vi "FTW-Socket-Bind.vi"(0 "FTW Endpoint":refnum<class "FTW-Socket.lvclass">, 5 "Remote Endpoint Address":string, 11 "error in":errorcluster) -> (4 "FTW Endpoint out":refnum<class "FTW-Socket.lvclass">, 6 "Actual Endpoint Address":string, 15 "error out":errorcluster)   [LabVIEW 2013, in "FTW-Socket.lvclass"]
uses:
  FTW-Socket.lvclass
  FTW-Socket.lvclass/FTW-Socket.ctl
panel:
  # "Inputs"
  # "Outputs"
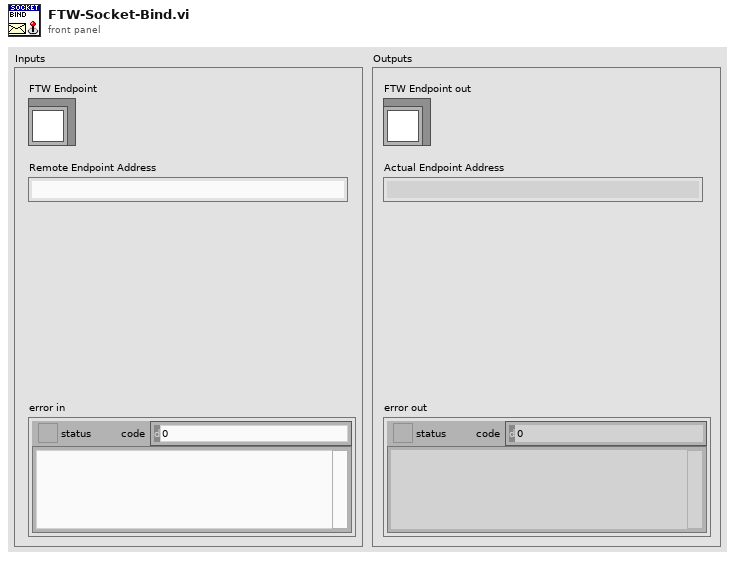
[diagram p1: front panel]
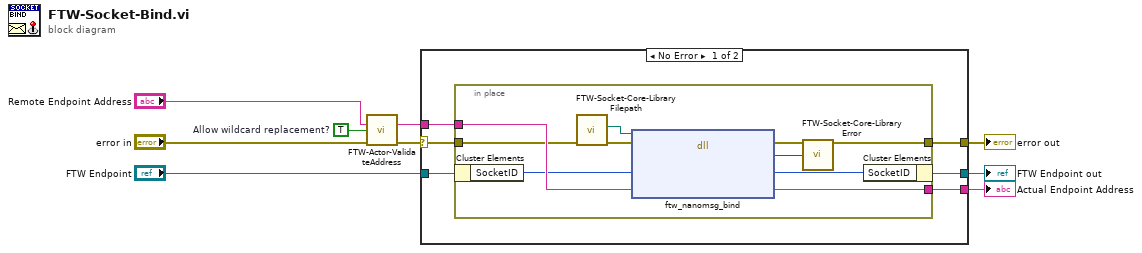
[diagram p0: block diagram]
diagram:
  w2 = TRUE  # Allow wildcard replacement?
  n1 = call "FTW-Actor-ValidateAddress.vi"("Address"="Remote Endpoint Address", "Allow wildcard replacement?"=w2, "error in"="error in") -> ("Sanitized Address"=w1:string, "error out"=w3:errorcluster)  [unwired: 10 in, 1 out]
  n2 = case shown="No Error" w3 {
    selector: w3 -> [w10 w26]
    tunnel: "FTW Endpoint" -> [w11 w27]
    tunnel: [w12 w26] -> w8
    tunnel: [w15 w27] -> w7
    tunnel: w1 -> [w14 _]
    tunnel: [w13 _] -> w6
    frame No Error {
      n3 = in-place {
        in-place-border: w10 -> [w21]
        in-place-border: w14 -> [w25]
        in-place-border: [w24] -> w13
        in-place-border: [w16] -> w12
        n4 = in-place-cluster #1(w11) -> ("SocketID"=w19:i64)
        n5 = call "FTW-Socket-Core-LibraryFilepath.vi"("error in"=w21) -> ("error out"=w20:errorcluster, "Library Filepath"=w22:path)  [unwired: 8 in, 1 out]
        n6 = dll-call lib="C:/Users/Jack/repo/ftw-master/Actor/src/Endpoint/Core/FTWLib-nanomsg32.dll" fn="ftw_nanomsg_bind"(path in=w22, error in=w20, "SocketID"=w19, "Address"=w25) -> (error out=w18:errorcluster, "Return Value"=w17:i64, "SocketID"=w23:i64, "Address"=w24:string)  [unwired: 1 in, 1 out]
        n7 = call "FTW-Socket-Core-LibraryError.vi"("error in"=w18, "Return Value"=w17) -> ("error out"=w16:errorcluster)  [unwired: 13 in]
        n8 = in-place-cluster #1("SocketID"=w23) -> (w15:refnum<class "FTW-Socket.lvclass">)
      }
    }
    frame Error {
    }
  }
  "error out" <- w8
  "FTW Endpoint out" <- w7
  "Actual Endpoint Address" <- w6
